vi "GenerateSignals(FPGA).vi"() -> ()   [LabVIEW 2011]
uses:
  <vilib>/rvi/interface/RandomDataEmulation/nirviRandomDataFPGAFIFO.vi
  <vilib>/rvi/interface/RandomDataEmulation/niFpgaRandomDataHandleErrors.vi
  <vilib>/rvi/DataTransferAndStorage/Container/XNode/niFpgaContainer.xnode
  <vilib>/rvi/interface/RandomDataEmulation/nirviRandomDataFpgaReadWriteTemplate.vi
panel:
  out "Timed Out?":bool
  in  "phase offset (periods)":fxp<+,32,0>=0.125
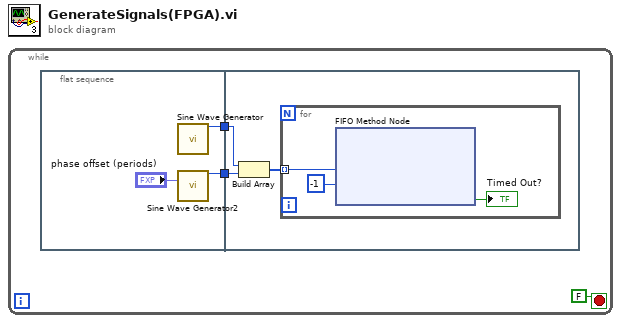
[diagram p0: block diagram]
diagram:
  n1 = while {
    stop <- FALSE stop-if-true
    n2 = flat-sequence {
      tunnel: [w5] -> w2
      tunnel: [w4] -> w1
      tunnel: w2 -> [w8]
      tunnel: w1 -> [w7]
      frame #0 {
        n3 = call "Sine Wave Generator"() -> ("sine out"=w5:i16)  [unwired: 15 in]
        n4 = call "Sine Wave Generator2"("phase offset (periods)"="phase offset (periods)") -> ("sine out"=w4:i16)  [unwired: 14 in]
      }
      frame #1 {
        n5 = Build Array(w8, w7) -> (w9:i16[])
        n6 = for {
          tunnel: w9 -> [w10] mode=indexing
          n7 = xnode ("FIFO Method Node")("Element"=w10, "Timeout"=-1) -> ("Timed Out?"=→"Timed Out?":bool)  [unwired: 1 in, 1 out]
        }
      }
    }
  }
